vi "V7310.Variable.Value.Get.vi"(6 "timeout ms (5000)":i32=5000, 8 "error in":errorcluster, 10 "Variable":string, 11 "Connection in":refnum<k5>) -> (0 "error out":errorcluster, 2 "Value":string, 3 "Connection out":refnum<k5>)   [LabVIEW 2016]
uses:
  LowLevel/V7310.Commands.ctl
panel:
  out "Data out":string
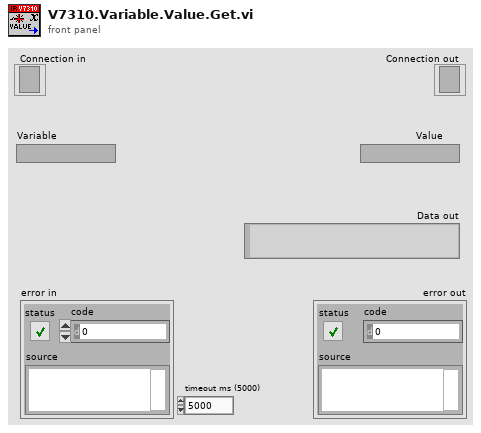
[diagram p1: front panel]
types:
  T1 = typedef "V7310.Commands.ctl" = enum16{"Start", "Stop", "GetStatus", "GetVarNames", "GetJobNames", "SetJob", "GetJob", "SetVars", "GetVars", "SetLayoutPosition", "SetRotation", "GetMessageID", "GetMessages", "ConfirmMessages", "DeleteMessages", "SetRTC", "GetRTC", "SetVarPosition", "SetIntensity", "GetIntensity", "SetStartTriggerDelay", "GetStartTriggerDelay", "SetStopTriggerDelay", "GetStopTriggerDelay", "SetConsecutiveTriggerDelay", "GetConsecutiveTriggerDelay", "SetMarkSpeed", "GetMarkSpeed"}
  T2 = typedef "V7310.ErrorLevels.ctl" = enum16{"OK", "Warning", "Error"}
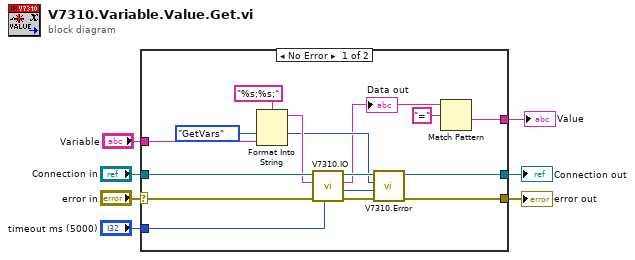
[diagram p0: block diagram]
diagram:
  n1 = case shown="No Error" "error in" {
    selector: "error in" -> [w19 w22]
    tunnel: "Connection in" -> [w20 w23]
    tunnel: [w21 w23] -> w6
    tunnel: "timeout ms (5000)" -> [w18 _]
    tunnel: [w13 w22] -> w3
    tunnel: "Variable" -> [w9 _]
    tunnel: [w8 _] -> w1
    frame No Error {
      w12 = V7310.Commands."GetVars" ("Cmd")
      n2 = Format Into String(format string="%s;%s;", w12, w9) -> (resulting string=w16:string)  [unwired: 2 in, 1 out]
      n3 = call "V7310.IO.vi"("timeout ms (5000)"=w18, "error in"=w19, "Data in"=w16, "Connection in"=w20) -> ("error out"=w14:errorcluster, "Error Level"=w15:T2, "Data out"=w11:string, "Connection out"=w21:refnum<k5>)  [unwired: 4 in]
      "Data out" <- w11
      n4 = call "V7310.Error.vi"("error in"=w14, "Error Level"=w15, "Cmd"=w12) -> ("error out"=w13:errorcluster)  [unwired: 8 in]
      n5 = Match Pattern(string=w11, regular expression="=") -> (after substring=w8:string)  [unwired: 1 in, 3 out]
    }
    frame Error {
    }
  }
  "Connection out" <- w6
  "error out" <- w3
  "Value" <- w1
